vi "EditParam1.vi"(9 "Index":u32, 10 "type":u16(ring)=2 items=["USB-CAN"=2, "USB-CAN2.0"=3], 11 "param":T1[](array[typedef]) {"ACR0" format="%x"}) -> (1 "Channels":u32[](array[numeric]), 2 "DevIndex":u32, 3 "param out":T1[](array[typedef]) {"ACR0" format="%x"})   [LabVIEW 2011]
doc: "ID=0x6004"
uses:
  Param.ctl
panel:
  out "label2":string="CAN参数"
  in  "AdvFilter":bool
  in  "AllChl":bool=TRUE
  in  "DevInd":u16(ring) caption="设备索引号:" items=["0", "1", "2", "3", "4", "5", "6", "7"]
  in  "Filter":u8(ring)=1 caption="滤波方式：" items=["接收所有类型"=1, "只收标准帧"=2, "只收扩展帧"=3]
  in  "Cancel":bool
  in  "OK":bool
  in  "channel":u16(ring) caption="选择CAN通道号:" items=["通道1", "通道2"]
  in  "屏蔽码":u32=4294967295 caption="过滤屏蔽码:" format="0x%08x"
  in  "验收码":u32=2147483648 caption="过滤验收码:" format="0x%08x"
  in  "工作模式:":u16(ring) items=["正常工作", "仅监帧听模式", "自测模试（环回模式）"]
  in  "BTR1":u8=28 caption="(HEX)" format="%02x"
  in  "BTR0":u8=1 caption="BTR0/1:" format="%02x"
  in  "br":u32(ring)=8 caption="波特率:" items=["Self Define", "5k bps", "10k bps", "20k bps", "40k bps", "50k bps", "80k bps", "100k bps", "125k bps", "200k bps", "250k bps", "400k bps", "500k bps", "666k bps", "800k bps", "1000k bps", "33.33k bps", "66.66k bps", "83.33k bps"]
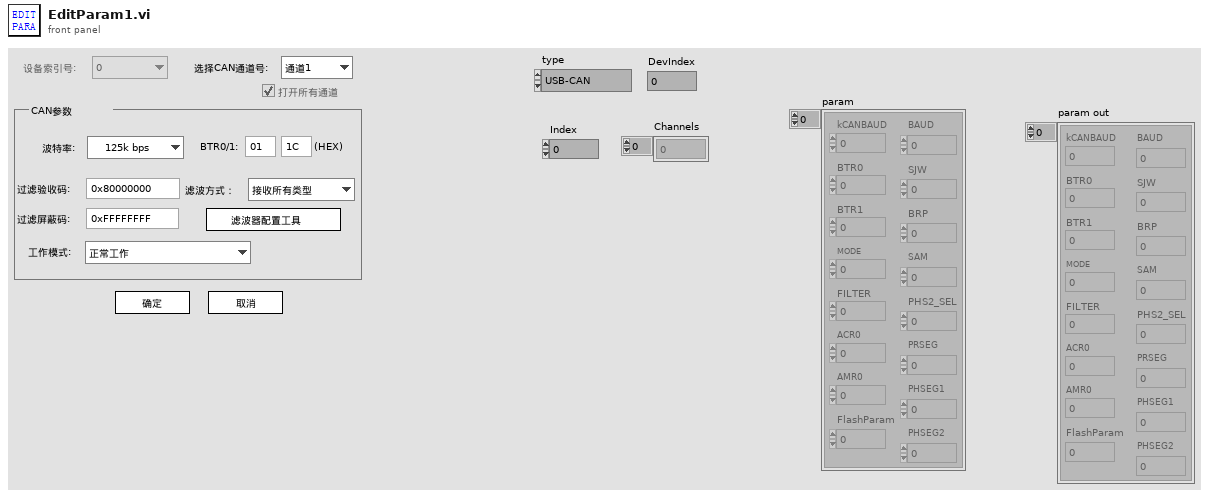
[diagram p1: front panel]
types:
  T1 = typedef "Param.ctl" = cluster{"kCANBAUD":u8, "BTR0":u8, "BTR1":u8, "MODE":u8, "FILTER":u8, "ACR0":u32, "AMR0":u32, "FlashParam":u32, "BAUD":u32, "SJW":u8, "BRP":u8, "SAM":u8, "PHS2_SEL":u8, "PRSEG":u8, "PHSEG1":u8, "PHSEG2":u8}
  T2 = enum8{"Enabled", "Disabled", "Disabled and Grayed Out"}
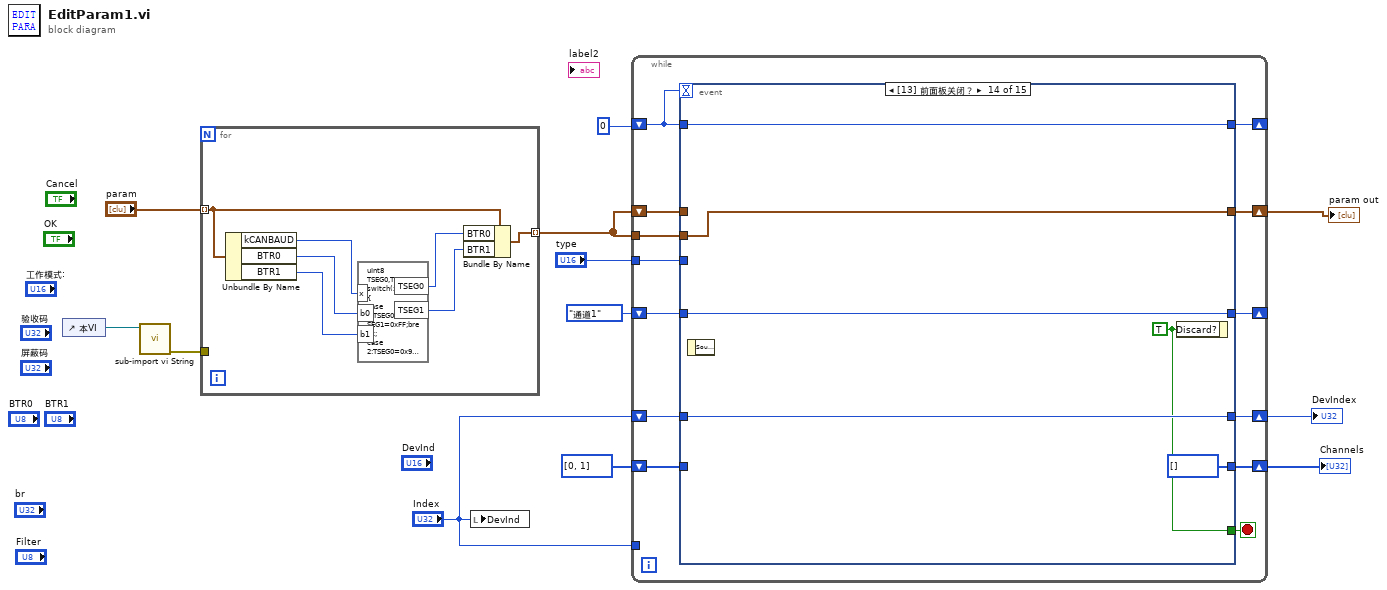
[diagram p0: block diagram]
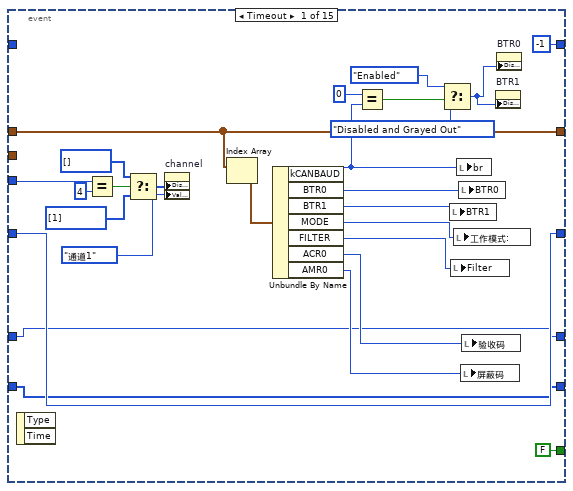
[diagram p2: hidden frame]
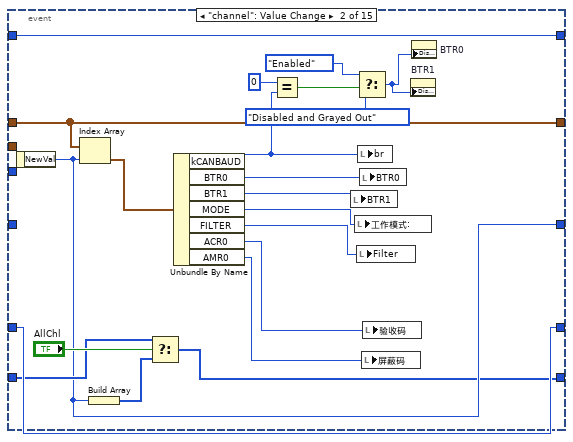
[diagram p3: hidden frame]
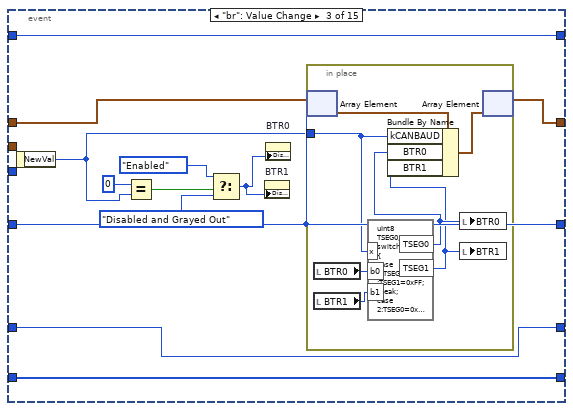
[diagram p4: hidden frame]
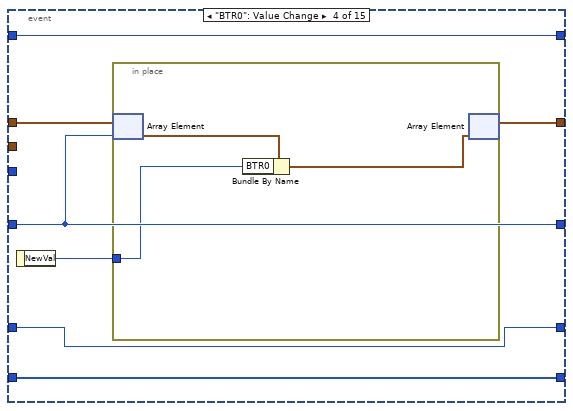
[diagram p5: hidden frame]
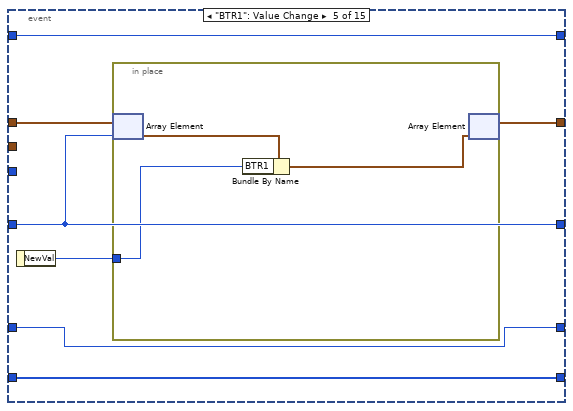
[diagram p6: hidden frame]
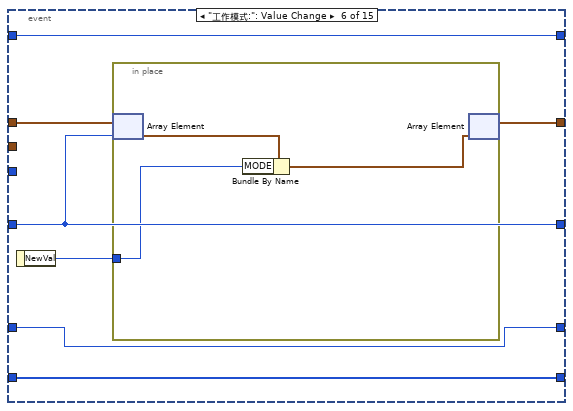
[diagram p7: hidden frame]
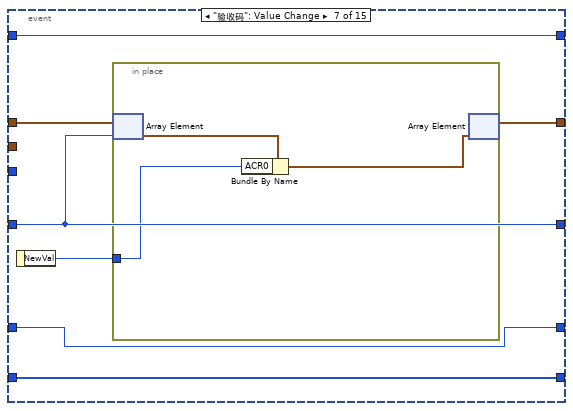
[diagram p8: hidden frame]
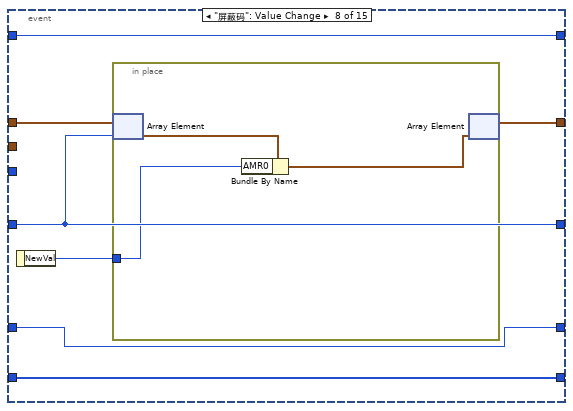
[diagram p9: hidden frame]
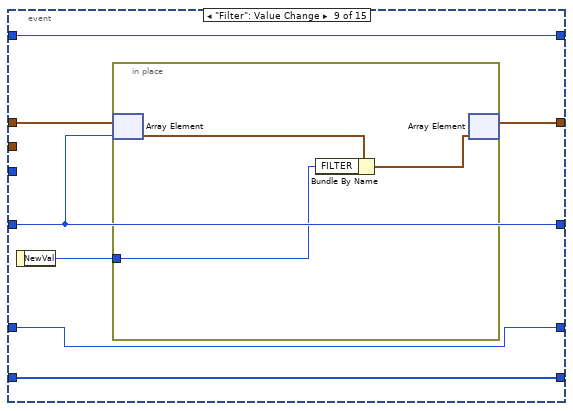
[diagram p10: hidden frame]
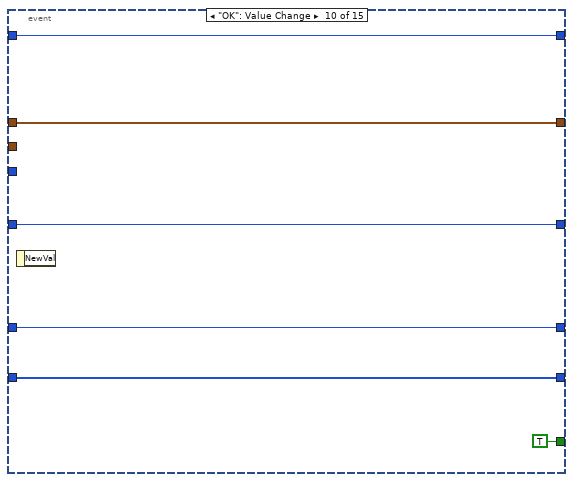
[diagram p11: hidden frame]
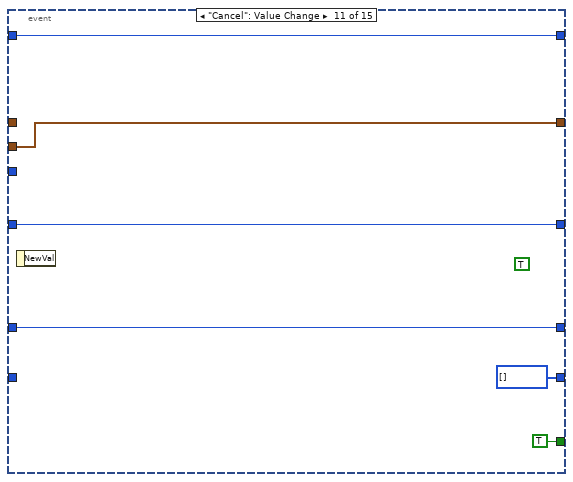
[diagram p12: hidden frame]
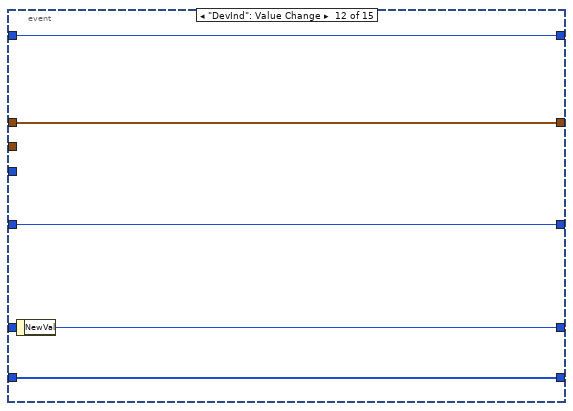
[diagram p13: hidden frame]
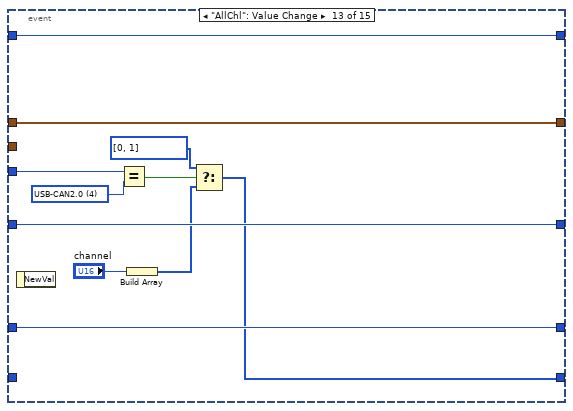
[diagram p14: hidden frame]
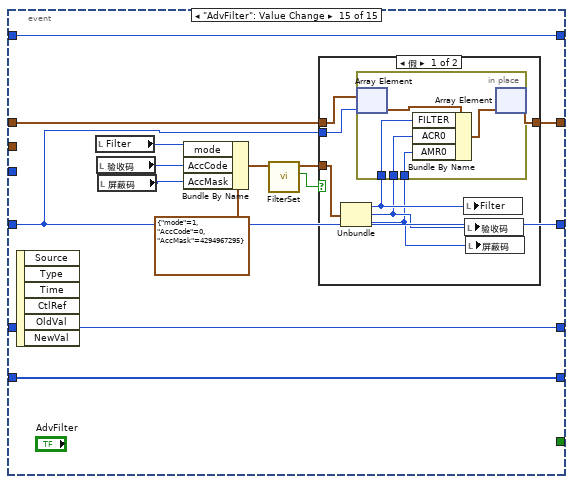
[diagram p15: hidden frame]
diagram:
  n1 = control-ref of="本VI"() -> (w2:refnum<vi>)
  n2 = call "sub-import vi String.vi"("vi ref"=w2) -> ("error out"=w1:errorcluster)  [unwired: 10 in]
  n3 = for {
    tunnel: "param" -> [w18] mode=indexing
    tunnel: [w17] -> w8 mode=indexing
    tunnel: w1 -> [_]
    n4 = Unbundle By Name(w18) -> ("kCANBAUD"=w19:u8, "BTR0"=w14:u8, "BTR1"=w13:u8)
    n5 = formula code="uInt8 TSEG0,TSEG1;\nswitch(x)\n{ \ncase 1:TSEG0=0x9F;TSEG1=0xFF;break;\ncase 2:TSEG0=0x9F;TSEG1=0xFF;break;\ncase 3:TSEG0=0x18;TSEG1=0x1c;break;\ncase 4:TSEG0=0x87;TSEG1=0xff;break;\ncase 5:TSEG0=0x09;TSEG1=0x1c;break;\ncase 6:TSEG0=0x83;TSEG1=0xff;break;\ncase 7:TSEG0=0x04;TSEG1=0x1c;break;\ncase 8:TSEG0=0x03;TSEG1=0x1c;break;\ncase 9:TSEG0=0x81;TSEG1=0xfa;break;\ncase 10:TSEG0=0x01;TSEG1=0x1c;break;\ncase 11:TSEG0=0x80;TSEG1=0xfa;break;\ncase 12:TSEG0=0x00;TSEG1=0x1c;break;\ncase 13:TSEG0=0x80;TSEG1=0xb6;break;\ncase 14:TSEG0=0x00;TSEG1=0x16;break;\ncase 15:TSEG0=0x00;TSEG1=0x14;break;\ncase 16:TSEG0=0x09;TSEG1=0x6F;break;\ncase 17:TSEG0=0x04;TSEG1=0x6F;break;\ncase 18:TSEG0=0x03;TSEG1=0x6F;break;\ndefault:TSEG0=b0;TSEG1=b1;break;\n}"("x"=w19, "b0"=w14, "b1"=w13) -> ("TSEG0"=w16:u8, "TSEG1"=w15:u8)
    n6 = Bundle By Name(cluster=w18, "BTR0"=w16, "BTR1"=w15) -> (w17:T1)
  }
  n7 = local write "DevInd"("Index") -> ()
  n8 = while {
    shift-right: [w30] -> w10
    shift-left: w8 -> [w31]
    shift-right: [w29] -> _
    shift-left: 0 -> [w28]
    tunnel: "type" -> [w27]
    shift-right: [w26] -> _
    shift-left: enum16{"通道1", "通道2"}."通道1" ("NewVal") -> [w25]
    tunnel: w8 -> [w24]
    shift-right: [w22] -> w7
    shift-left: "Index" -> [w23]
    shift-right: [w20] -> w5
    shift-left: u32[] [0, 1] ("Channels") -> [w21]
    tunnel: "Index" -> [_]
    stop <- w32 stop-if-true
    n9 = event shown="[13] 前面板关闭？" {
      selector: _ -> [_ _ _ _ _ _ _ _ _ _ _ _ _ _ _]
      dyn-events: _ -> [_ _ _ _ _ _ _ _ _ _ _ _ _ _ _]
      timeout: w28 -> [_ _ _ _ _ _ _ _ _ _ _ _ _ _ _]
      tunnel: [FALSE _ _ _ _ _ _ _ _ TRUE TRUE _ _ w187 _] -> w32
      tunnel: w31 -> [w49 w78 w85 w104 w114 w124 w134 w144 w154 w164 _ w175 w186 _ w195]
      tunnel: [w49 w78 w83 w102 w112 w122 w132 w142 w153 w164 w167 w175 w186 w190 w194] -> w30
      tunnel: [-1 w79 w91 w105 w115 w125 w135 w145 w155 w163 w170 w174 w185 w192 w205] -> w29
      tunnel: w28 -> [_ w79 w91 w105 w115 w125 w135 w145 w155 w163 w170 w174 w185 w192 w205]
      tunnel: w27 -> [w56 _ _ _ _ _ _ _ _ _ _ _ w182 _ _]
      tunnel: [w36 w61 w84 w101 w111 w121 w131 w141 w152 w162 w169 w173 w184 w191 w193] -> w26
      tunnel: w25 -> [w36 _ w84 w101 w111 w121 w131 w141 w152 w162 w169 w173 w184 w191 w193]
      tunnel: w24 -> [_ _ _ _ _ _ _ _ _ _ w167 _ _ w190 _]
      tunnel: w23 -> [w34 w64 w81 w100 w110 w120 w130 w140 w150 w160 w166 _ w183 w189 w204]
      tunnel: [w34 w64 w81 w100 w110 w120 w130 w140 w150 w160 w166 w172 w183 w189 w204] -> w22
      tunnel: w21 -> [w33 w62 w80 w99 w109 w119 w129 w139 w149 w159 _ w171 _ _ w203]
      tunnel: [w33 w59 w80 w99 w109 w119 w129 w139 w149 w159 u32[] [] ("Channels") w171 w176 u32[] [] ("Channels") w203] -> w20
      event Timeout {
        n10 = event-data() -> ()  [unwired: 1 in, 2 out]
        n11 = Equal?(x=w56, y=u16 4) -> (x = y?=w54:bool)
        n12 = Select(t=i32[] [] ("禁用项[]"), s=w54, f=i32[] [1] ("禁用项[]")) -> (s? t:f=w51:i32[])
        n13 = property on="channel" class="Ring (严格)"("Disabled Items []"=w51, "Value"=enum16{"通道1", "通道2"}."通道1" ("channel")) -> ()  [unwired: 2 in, 2 out]
        n14 = Index Array(array=w49) -> (element=w48:T1)  [unwired: 1 in]
        n15 = Unbundle By Name(w48) -> ("kCANBAUD"=w42:u8, "BTR0"=w47:u8, "BTR1"=w46:u8, "MODE"=w45:u8, "FILTER"=w35:u8, "ACR0"=w44:u32, "AMR0"=w43:u32)
        n16 = Equal?(x=u8 0, y=w42) -> (x = y?=w38:bool)
        n17 = Select(t=T2."Enabled" ("禁用"), s=w38, f=T2."Disabled and Grayed Out") -> (s? t:f=w37:T2)
        n18 = local write "BTR1"(w46) -> ()
        n19 = local write "Filter"(w35) -> ()
        n20 = local write "工作模式:"(w45) -> ()
        n21 = local write "br"(w42) -> ()
        n22 = local write "BTR0"(w47) -> ()
        n23 = local write "屏蔽码"(w43) -> ()
        n24 = local write "验收码"(w44) -> ()
        n25 = property on="BTR1" class="DigNum (严格)"("DisabledEnum"=w37) -> ()  [unwired: 2 in, 2 out]
        n26 = property on="BTR0" class="DigNum (严格)"("DisabledEnum"=w37) -> ()  [unwired: 2 in, 2 out]
      }
      event "channel": Value Change {
        n27 = event-data() -> ("NewVal"=w61:u16)  [unwired: 1 in]
        n28 = Index Array(array=w78, index=w61) -> (element=w72:T1)
        n29 = Build Array(w61) -> (w60:u16[])
        n30 = Select(t=w62, s="AllChl", f=w60) -> (s? t:f=w59:u32[])
        n31 = Unbundle By Name(w72) -> ("kCANBAUD"=w66:u8, "BTR0"=w77:u8, "BTR1"=w76:u8, "MODE"=w75:u8, "FILTER"=w65:u8, "ACR0"=w74:u32, "AMR0"=w73:u32)
        n32 = Equal?(x=u8 0, y=w66) -> (x = y?=w68:bool)
        n33 = local write "BTR1"(w76) -> ()
        n34 = local write "工作模式:"(w75) -> ()
        n35 = Select(t=T2."Enabled" ("禁用"), s=w68, f=T2."Disabled and Grayed Out") -> (s? t:f=w67:T2)
        n36 = local write "Filter"(w65) -> ()
        n37 = local write "br"(w66) -> ()
        n38 = local write "BTR0"(w77) -> ()
        n39 = local write "屏蔽码"(w73) -> ()
        n40 = local write "验收码"(w74) -> ()
        n41 = property on="BTR1" class="DigNum (严格)"("DisabledEnum"=w67) -> ()  [unwired: 2 in, 2 out]
        n42 = property on="BTR0" class="DigNum (严格)"("DisabledEnum"=w67) -> ()  [unwired: 2 in, 2 out]
      }
      event "br": Value Change {
        n43 = event-data() -> ("NewVal"=w82:u32)  [unwired: 1 in]
        n44 = Equal?(x=u8 0, y=w82) -> (x = y?=w89:bool)
        n45 = Select(t=T2."Enabled" ("禁用"), s=w89, f=T2."Disabled and Grayed Out") -> (s? t:f=w88:T2)
        n46 = property on="BTR1" class="DigNum (严格)"("DisabledEnum"=w88) -> ()  [unwired: 2 in, 2 out]
        n47 = property on="BTR0" class="DigNum (严格)"("DisabledEnum"=w88) -> ()  [unwired: 2 in, 2 out]
        n48 = in-place {
          in-place-border: w82 -> [w96]
          n49 = in-place-array #1(w85, w84) -> (w98:T1)
          n50 = local read "BTR0"() -> (w93:u8)
          n51 = local read "BTR1"() -> (w92:u8)
          n52 = formula code="uInt8 TSEG0,TSEG1;\nswitch(x)\n{ \ncase 1:TSEG0=0x9F;TSEG1=0xFF;break;\ncase 2:TSEG0=0x9F;TSEG1=0xFF;break;\ncase 3:TSEG0=0x18;TSEG1=0x1c;break;\ncase 4:TSEG0=0x87;TSEG1=0xff;break;\ncase 5:TSEG0=0x09;TSEG1=0x1c;break;\ncase 6:TSEG0=0x83;TSEG1=0xff;break;\ncase 7:TSEG0=0x04;TSEG1=0x1c;break;\ncase 8:TSEG0=0x03;TSEG1=0x1c;break;\ncase 9:TSEG0=0x81;TSEG1=0xfa;break;\ncase 10:TSEG0=0x01;TSEG1=0x1c;break;\ncase 11:TSEG0=0x80;TSEG1=0xfa;break;\ncase 12:TSEG0=0x00;TSEG1=0x1c;break;\ncase 13:TSEG0=0x80;TSEG1=0xb6;break;\ncase 14:TSEG0=0x00;TSEG1=0x16;break;\ncase 15:TSEG0=0x00;TSEG1=0x14;break;\ncase 16:TSEG0=0x09;TSEG1=0x6F;break;\ncase 17:TSEG0=0x04;TSEG1=0x6F;break;\ncase 18:TSEG0=0x03;TSEG1=0x6F;break;\ndefault:TSEG0=b0;TSEG1=b1;break;\n}"("x"=w96, "b0"=w93, "b1"=w92) -> ("TSEG0"=w95:u8, "TSEG1"=w94:u8)
          n53 = Bundle By Name(cluster=w98, "kCANBAUD"=w96, "BTR0"=w95, "BTR1"=w94) -> (w97:T1)
          n54 = local write "BTR0"(w95) -> ()
          n55 = local write "BTR1"(w94) -> ()
          n56 = in-place-array #1(w97) -> (w83:T1[])  [unwired: 1 out]
        }
      }
      event "BTR0": Value Change {
        n57 = event-data() -> ("NewVal"=w103:u8)  [unwired: 1 in]
        n58 = in-place {
          in-place-border: w103 -> [w107]
          n59 = in-place-array #2(w104, w101) -> (w108:T1)
          n60 = Bundle By Name(cluster=w108, "BTR0"=w107) -> (w106:T1)
          n61 = in-place-array #2(w106) -> (w102:T1[])  [unwired: 1 out]
        }
      }
      event "BTR1": Value Change {
        n62 = event-data() -> ("NewVal"=w113:u8)  [unwired: 1 in]
        n63 = in-place {
          in-place-border: w113 -> [w117]
          n64 = in-place-array #3(w114, w111) -> (w118:T1)
          n65 = Bundle By Name(cluster=w118, "BTR1"=w117) -> (w116:T1)
          n66 = in-place-array #3(w116) -> (w112:T1[])  [unwired: 1 out]
        }
      }
      event "工作模式:": Value Change {
        n67 = event-data() -> ("NewVal"=w123:u16)  [unwired: 1 in]
        n68 = in-place {
          in-place-border: w123 -> [w127]
          n69 = in-place-array #4(w124, w121) -> (w128:T1)
          n70 = Bundle By Name(cluster=w128, "MODE"=w127) -> (w126:T1)
          n71 = in-place-array #4(w126) -> (w122:T1[])  [unwired: 1 out]
        }
      }
      event "验收码": Value Change {
        n72 = event-data() -> ("NewVal"=w133:u32)  [unwired: 1 in]
        n73 = in-place {
          in-place-border: w133 -> [w137]
          n74 = in-place-array #5(w134, w131) -> (w138:T1)
          n75 = Bundle By Name(cluster=w138, "ACR0"=w137) -> (w136:T1)
          n76 = in-place-array #5(w136) -> (w132:T1[])  [unwired: 1 out]
        }
      }
      event "屏蔽码": Value Change {
        n77 = event-data() -> ("NewVal"=w143:u32)  [unwired: 1 in]
        n78 = in-place {
          in-place-border: w143 -> [w147]
          n79 = in-place-array #6(w144, w141) -> (w148:T1)
          n80 = Bundle By Name(cluster=w148, "AMR0"=w147) -> (w146:T1)
          n81 = in-place-array #6(w146) -> (w142:T1[])  [unwired: 1 out]
        }
      }
      event "Filter": Value Change {
        n82 = event-data() -> ("NewVal"=w151:u8)  [unwired: 1 in]
        n83 = in-place {
          in-place-border: w151 -> [w156]
          n84 = in-place-array #7(w154, w152) -> (w158:T1)
          n85 = Bundle By Name(cluster=w158, "FILTER"=w156) -> (w157:T1)
          n86 = in-place-array #7(w157) -> (w153:T1[])  [unwired: 1 out]
        }
      }
      event "OK": Value Change {
        n87 = event-data() -> ()  [unwired: 1 in, 1 out]
      }
      event "Cancel": Value Change {
        (unwired) TRUE
        n88 = event-data() -> ()  [unwired: 1 in, 1 out]
      }
      event "DevInd": Value Change {
        n89 = event-data() -> ("NewVal"=w172:u16)  [unwired: 1 in]
      }
      event "AllChl": Value Change {
        w181 = u16 4 items=["USB-CAN"=3, "USB-CAN2.0"=4] ("type")
        n90 = event-data() -> ()  [unwired: 1 in, 1 out]
        n91 = Equal?(x=w182, y=w181) -> (x = y?=w180:bool)
        n92 = Build Array("channel") -> (w177:u16[])
        n93 = Select(t=u32[] [0, 1] ("Channels"), s=w180, f=w177) -> (s? t:f=w176:u32[])
      }
      event Panel Close? {
        w187 = TRUE ("放弃？")
        n94 = event-data() -> ()  [unwired: 1 in, 1 out]
        n95 = event-data("Discard?"=w187) -> ()  [unwired: 1 in, 1 out]
      }
      event "AdvFilter": Value Change {
        n96 = event-data() -> ()  [unwired: 1 in, 6 out]
        n97 = local read "Filter"() -> (w200:u8)
        n98 = local read "验收码"() -> (w199:u32)
        n99 = local read "屏蔽码"() -> (w198:u32)
        n100 = Bundle By Name(cluster=cluster{"mode":u8, "AccCode":u32, "AccMask":u32} {"mode"=1, "AccCode"=0, "AccMask"=4294967295} ("ParamIn"), "mode"=w200, "AccCode"=w199, "AccMask"=w198) -> (w201:cluster{"mode":u8, "AccCode":u32, "AccMask":u32})
        n101 = call "FilterSet.vi"("ParamIn"=w201) -> ("Cancel？"=w197:bool, "ParamOut"=w196:cluster{"mode":u8, "AccCode":u32, "AccMask":u32})  [unwired: 8 in, 1 out]
        n102 = case shown="假" w197 {
          tunnel: w196 -> [w212 _]
          tunnel: w195 -> [w211 w218]
          tunnel: [w209 w218] -> w194
          tunnel: w193 -> [w210 _]
          frame False {
            n103 = Unbundle(w212) -> ("mode"=w208:u8, "AccCode"=w207:u32, "AccMask"=w206:u32)
            n104 = in-place {
              in-place-border: w208 -> [w216]
              in-place-border: w207 -> [w214]
              in-place-border: w206 -> [w213]
              n105 = in-place-array #8(w211, w210) -> (w217:T1)
              n106 = Bundle By Name(cluster=w217, "FILTER"=w216, "ACR0"=w214, "AMR0"=w213) -> (w215:T1)
              n107 = in-place-array #8(w215) -> (w209:T1[])  [unwired: 1 out]
            }
            n108 = local write "Filter"(w208) -> ()
            n109 = local write "验收码"(w207) -> ()
            n110 = local write "屏蔽码"(w206) -> ()
          }
          frame True {
          }
        }
      }
    }
  }
  "param out" <- w10
  "DevIndex" <- w7
  "Channels" <- w5
